vi "Tabelle initialisieren.vi"(9 "Neue Tabelle":T1) -> (1 "Tabelle":string[][](array[string]))   [LabVIEW 2020, in "Linearisierung v2.lvlib"]
uses:
  Linearisierung v2.lvlib
  Eingabetabelle.ctl
  Allgemein/allgemeine Sub-VIs.lvlib
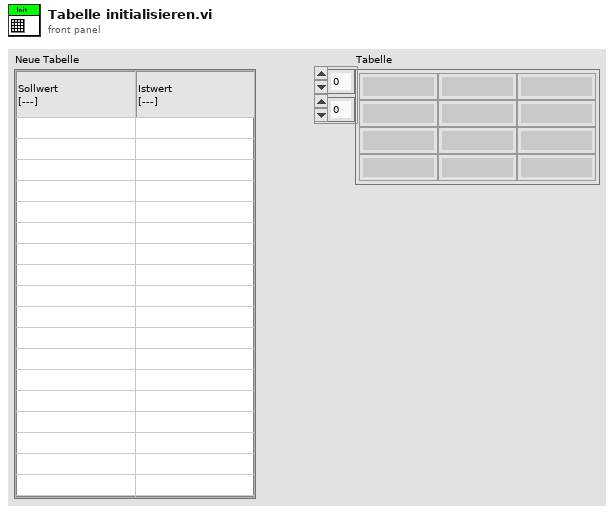
[diagram p1: front panel]
types:
  T1 = typedef "Linearisierung v2.lvlib/Eingabetabelle.ctl" = string[][]
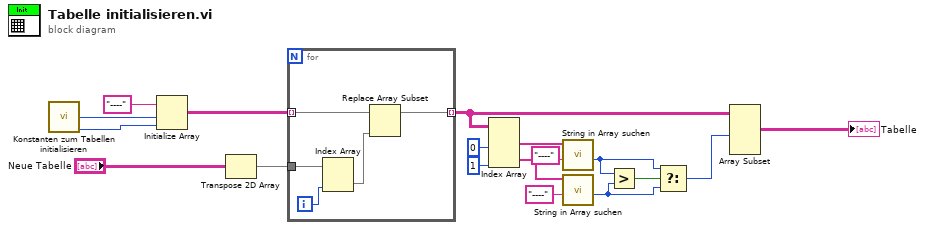
[diagram p0: block diagram]
diagram:
  n1 = call "Konstanten zum Tabellen initialisieren.vi"() -> ("Anzahl Tabellenzeilen"=w2:i32, "Anzahl Tabellenspalten"=w1:i32)  [unwired: 13 in, 1 out]
  n2 = Initialize Array("----", w2, w1) -> (w14:string[][])
  n3 = Transpose 2D Array(2D array="Neue Tabelle") -> (transposed array=w10:T1)
  n4 = for {
    tunnel: w14 -> [w23] mode=indexing
    tunnel: w10 -> [w22]
    tunnel: [w19] -> w12 mode=indexing
    i -> [w21]
    n5 = Index Array(array=w22, index (col)=w21) -> (element=w20:string[])  [unwired: 1 in]
    n6 = Replace Array Subset(array=w23, new element=w20) -> (w19:string[])  [unwired: 1 in]
  }
  n7 = Index Array(array=w12, index (col) #1=0 ("Deaktivierter Index (Spalte)"), index (col) #2=1 ("Index (Spalte)")) -> (element #1=w16:string[], element #2=w3:string[])  [unwired: 2 in]
  n8 = call "String in Array suchen.vi"("Nach String/Zeichen suchen (-)"="----", "String-Array"=w16) -> ("Index"=w6:i32)  [unwired: 7 in, 2 out]
  n9 = call "String in Array suchen.vi"("Nach String/Zeichen suchen (-)"="----", "String-Array"=w3) -> ("Index"=w5:i32)  [unwired: 7 in, 2 out]
  n10 = Greater?(x=w6, y=w5) -> (0:w7:bool)
  n11 = Select(t=w6, s=w7, f=w5) -> (s? t:f=w4:i32)
  n12 = Array Subset(array=w12, length (row)=w4) -> (→"Tabelle":string[][])  [unwired: 3 in]
